vi "Check Empty JSON Dict.vi"(11 "JSON in":string) -> (3 "JSON out":string)   [LabVIEW 2020, in "wamplv.lvlib" / "Utils.lvclass"]
uses:
  Utils.lvclass
  Utils.lvclass/Utils.ctl
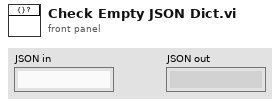
[diagram p1: front panel]
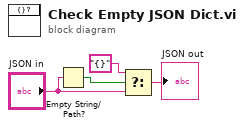
[diagram p0: block diagram]
diagram:
  n1 = Empty String/Path?(string/path="JSON in") -> (empty?=w4:bool)
  n2 = Select(t="{}" ("f"), s=w4, f="JSON in") -> (s? t:f=→"JSON out":string)
